vi "CH3_Save_Header_Python.vi"() -> ()   [LabVIEW 2018]
uses:
  RxTx/RxTx.lvclass
  Save Image/Save Image.lvclass
  Channel/Channel.lvclass
panel:
  out "error out":errorcluster
  in  "Save Image out":refnum<class "Save Image.lvclass">
  in  "RxTx.lvclass":refnum<class "RxTx.lvclass">
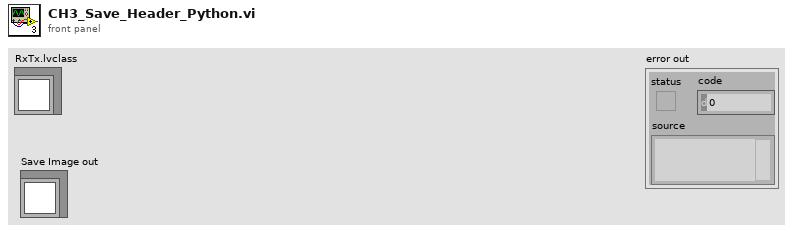
[diagram p1: front panel]
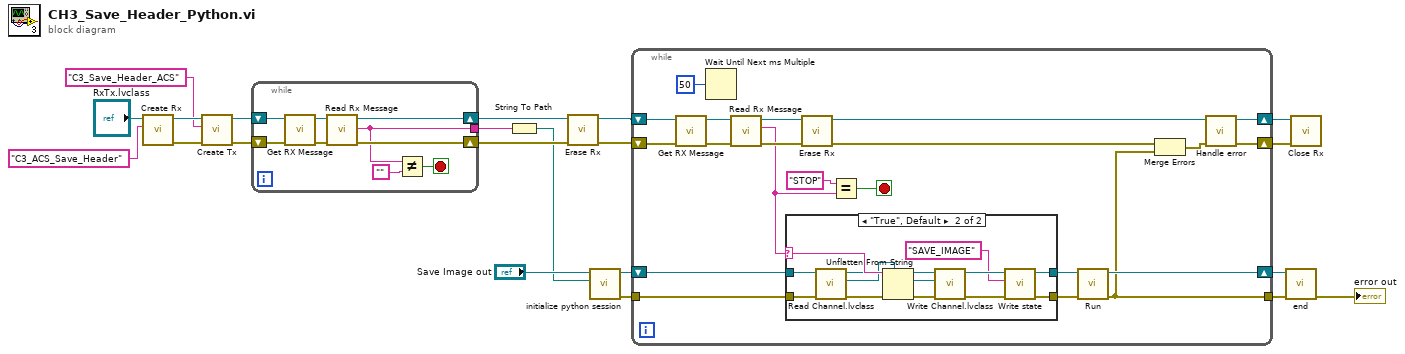
[diagram p0: block diagram]
diagram:
  n1 = call "Create Rx.vi"("Reader Name"="C3_ACS_Save_Header", "RxTx in"="RxTx.lvclass") -> ("error out"=w6:errorcluster, "RxTx out"=w9:refnum<class "RxTx.lvclass">)  [unwired: 8 in]
  n2 = call "Create Tx.vi"("error in (no error)"=w6, "Writer Name"="C3_Save_Header_ACS" ("Reader Name"), "RxTx in"=w9) -> ("error out"=w7:errorcluster, "RxTx out"=w8:refnum<class "RxTx.lvclass">)  [unwired: 7 in]
  n3 = while {
    shift-right: [w28] -> w16
    shift-left: w7 -> [w30]
    shift-right: [w27] -> w13
    shift-left: w8 -> [w25]
    tunnel: [w22] -> w11
    stop <- w23 stop-if-true
    n4 = call "Get RX Message.vi"("error in (no error)"=w30, "RxTx in"=w25) -> ("error out"=w29:errorcluster, "RxTx out"=w26:refnum<class "RxTx.lvclass">)  [unwired: 8 in]
    n5 = call "Read Rx Message.vi"("error in (no error)"=w29, "RxTx in"=w26) -> ("error out"=w28:errorcluster, "Rx Message"=w22:string, "RxTx out"=w27:refnum<class "RxTx.lvclass">)  [unwired: 7 in]
    n6 = Not Equal?(x=w22, y="") -> (x != y?=w23:bool)
  }
  n7 = String To Path(string=w11) -> (path=w12:path)
  n8 = call "Erase Rx.vi"("error in (no error)"=w16, "RxTx in"=w13) -> ("error out"=w15:errorcluster, "RxTx out"=w14:refnum<class "RxTx.lvclass">)  [unwired: 8 in]
  n9 = call "initialize python session.vi"("Optional Path to Python.exe"=w12, "Save Image in"="Save Image out") -> ("error out"=w3:errorcluster, "Save Image out"=w19:refnum<class "Save Image.lvclass">)  [unwired: 8 in]
  n10 = while {
    shift-right: [w35] -> w4
    shift-left: w14 -> [w51]
    shift-right: [w43] -> w17
    shift-left: w19 -> [w44]
    shift-right: [w34] -> w1
    shift-left: w15 -> [w50]
    tunnel: w3 -> [w37]
    tunnel: [w36] -> w2
    stop <- w38 stop-if-true
    n11 = call "Get RX Message.vi"("error in (no error)"=w50, "RxTx in"=w51) -> ("error out"=w48:errorcluster, "RxTx out"=w49:refnum<class "RxTx.lvclass">)  [unwired: 8 in]
    n12 = Wait Until Next ms Multiple(millisecond multiple=u32 50) -> ()  [unwired: 1 out]
    n13 = call "Read Rx Message.vi"("error in (no error)"=w48, "RxTx in"=w49) -> ("error out"=w41:errorcluster, "Rx Message"=w39:string, "RxTx out"=w42:refnum<class "RxTx.lvclass">)  [unwired: 7 in]
    n14 = case shown="\"True\", Default" w39 {
      selector: w39 -> [_ w66]
      tunnel: [w53 w57] -> w46
      tunnel: [w52 w55] -> w45
      tunnel: w37 -> [w52 w64]
      tunnel: w44 -> [w53 w65]
      frame "", "STOP" {
      }
      frame "True", Default {
        n15 = call-dynamic "Read Channel.lvclass.vi"("error in (no error)"=w64, "Save Image in"=w65) -> ("error out"=w63:errorcluster, "Channel.lvclass"=w60:refnum<class "Channel.lvclass">, "Save Image out"=w61:refnum<class "Save Image.lvclass">)  [unwired: 7 in]
        n16 = Unflatten From String(type=w60, binary string=w66, error in (no error)=w63) -> (value=w59:refnum<class "Channel.lvclass">, error out=w62:errorcluster)  [unwired: 2 in, 1 out]
        n17 = call-dynamic "Write Channel.lvclass.vi"("error in (no error)"=w62, "Channel.lvclass"=w59, "Save Image in"=w61) -> ("error out"=w56:errorcluster, "Save Image out"=w58:refnum<class "Save Image.lvclass">)  [unwired: 7 in]
        n18 = call "Write state.vi"("error in (no error)"=w56, "String"="SAVE_IMAGE" ("Reader Name"), "Save Image in"=w58) -> ("error out"=w55:errorcluster, "Save Image out"=w57:refnum<class "Save Image.lvclass">)  [unwired: 7 in]
      }
    }
    n19 = call "Erase Rx.vi"("error in (no error)"=w41, "RxTx in"=w42) -> ("error out"=w32:errorcluster, "RxTx out"=w33:refnum<class "RxTx.lvclass">)  [unwired: 8 in]
    n20 = Equal?(x="STOP" ("Reader Name"), y=w39) -> (x = y?=w38:bool)
    n21 = call "Run.vi"("error in (no error)"=w45, "Save Image in"=w46) -> ("error out"=w36:errorcluster, "Save Image out"=w43:refnum<class "Save Image.lvclass">)  [unwired: 8 in]
    n22 = Merge Errors(w32, w36) -> (w31:errorcluster)
    n23 = call "Handle error.vi"("error in (no error)"=w31, "RxTx in"=w33) -> ("error out"=w34:errorcluster, "RxTx out"=w35:refnum<class "RxTx.lvclass">)  [unwired: 8 in]
  }
  n24 = call "end.vi"("error in (no error)"=w2, "Save Image in"=w17) -> ("error out"=→"error out":errorcluster)  [unwired: 8 in, 1 out]
  n25 = call "Close Rx.vi"("error in (no error)"=w1, "RxTx in"=w4) -> ()  [unwired: 8 in, 2 out]
